vi "fgv_GNSS-Ntrip_ctrl-refs.vi"(7 "cmd":T2, 11 "ref":T1) -> (3 "ref 2":T1)   [LabVIEW 2019]
uses:
  Ctrl/cmd_common.ctl
  Ctrl/GNSS-Ntrip ref.ctl
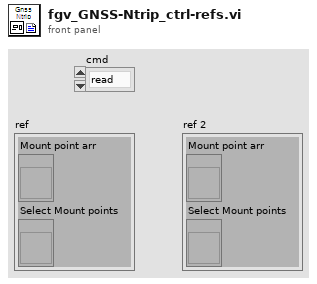
[diagram p1: front panel]
types:
  T1 = typedef "GNSS-Ntrip ref.ctl" = cluster{"Mount point arr":refnum<vi>, "Select Mount points":refnum<vi>}
  T2 = typedef "cmd_common.ctl" = enum16{"read", "write"}
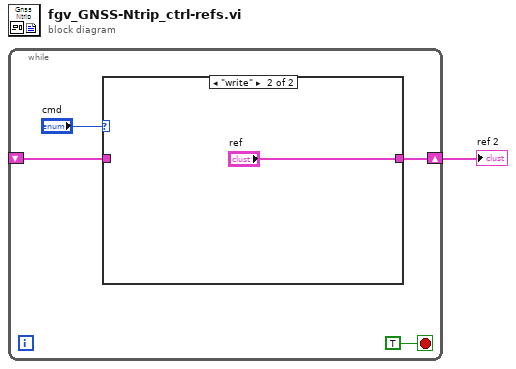
[diagram p0: block diagram]
diagram:
  n1 = while {
    shift-right: [w3] -> w1
    shift-left: _ -> [w2]
    stop <- TRUE stop-if-true
    n2 = case shown="\"write\"" "cmd" {
      tunnel: [w6 "ref"] -> w3
      tunnel: w2 -> [w6 _]
      frame "read", Default {
      }
      frame "write" {
      }
    }
  }
  "ref 2" <- w1
